vi "Execute.vi"(8 "error in (no error)":errorcluster, 10 "User Events in":refnum<class "User Events.lvclass">, 11 "Controller in":refnum<class "Controller.lvclass">) -> (0 "error out":errorcluster, 3 "Controller out":refnum<class "Controller.lvclass">)   [LabVIEW 2016, in "Controller.lvclass"]
uses:
  Controller.lvclass
  User Events/User Events.lvclass
  Typedefs/StateTypes.ctl
  User Events/User Events.lvclass/User Events.ctl
  Commands/Command/Command.lvclass
  Typedefs/HPMT_Typedefs.lvlib
  Model/Model/Model.lvclass
  Model/Boot Loader/Boot Loader.lvclass
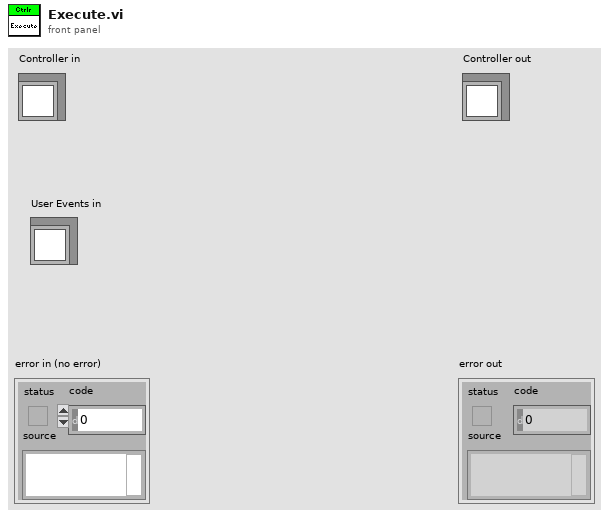
[diagram p1: front panel]
types:
  T1 = typedef "HPMT_Typedefs.lvlib/StateTypes.ctl" = enum16{"Offline State", "Fault State", "Standby State", "Disabled State", "Enabled State", "Wait For User Input State", "Test Actuator State", "Manual State"}
  T2 = typedef "HPMT_Typedefs.lvlib/Subscribe Data Events.ctl" = cluster{"Command":refnum<user-event>}
  T3 = typedef "HPMT_Typedefs.lvlib/Publish Data Events.ctl" = cluster{"State":refnum<user-event>, "ErrorCode":refnum<user-event>, "Scan Progress":refnum<user-event>, "All Test Status":refnum<user-event>, "ActuatorData":refnum<user-event>, "Test Settings":refnum<user-event>, "Stop Constant Query":refnum<user-event>}
  T4 = cluster{"Event Registration Refnum":refnum<event-registration>, "Event Registration Refnum":refnum<event-registration>}
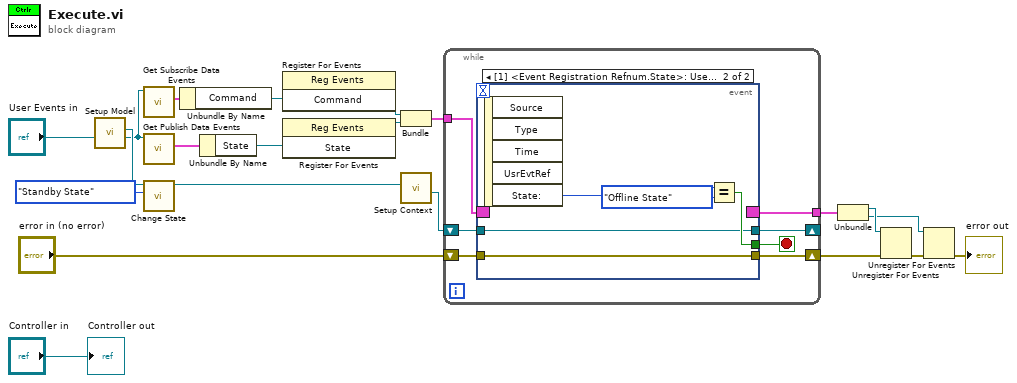
[diagram p0: block diagram]
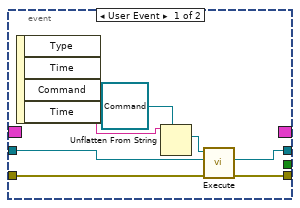
[diagram p2: hidden frame]
diagram:
  n1 = call "Setup Model.vi"("User Events in"="User Events in") -> ("User Events out"=w11:refnum<class "User Events.lvclass">, "Model out"=w16:refnum<class "Model.lvclass">)  [unwired: 7 in, 2 out]
  n2 = call "Get Subscribe Data Events.vi"("UserEvents in"=w11) -> ("Subscribe Data Events"=w20:T2)  [unwired: 9 in, 1 out]
  n3 = call "Get Publish Data Events.vi"("UserEvents in"=w11) -> ("Publish Data Events"=w10:T3)  [unwired: 9 in, 1 out]
  n4 = call "Change State.vi"("State Types"=StateTypes."Standby State" ("State:"), "Model in"=w16) -> ("Model out"=w15:refnum<class "Model.lvclass">)  [unwired: 8 in, 1 out]
  n5 = Unbundle By Name(w20) -> ("Command"=w18:refnum<user-event>)
  n6 = Unbundle By Name(w10) -> ("State"=w9:refnum<user-event>)
  n7 = register-events(w18) -> (reference out=w8:refnum<event-registration>)  [unwired: 2 in, 1 out]
  n8 = register-events(w9) -> (reference out=w7:refnum<event-registration>)  [unwired: 2 in, 1 out]
  n9 = Bundle("Event Registration Refnum"=w8, "Event Registration Refnum"=w7) -> (w6:T4)  [unwired: 1 in]
  n10 = call "Setup Context.vi"("Model in"=w15) -> ("Context out"=w14:refnum<class "Context.lvclass">)  [unwired: 8 in, 2 out]
  n11 = while {
    shift-right: [w27] -> w19
    shift-left: "error in (no error)" -> [w24]
    shift-right: [w26] -> _
    shift-left: w14 -> [w28]
    tunnel: w6 -> [w23]
    tunnel: [w22] -> w5
    stop <- w25 stop-if-true
    n12 = event shown="[1] <Event Registration Refnum.State>: User Event" {
      selector: w23 -> [_ _]
      dyn-events: [_ _] -> w22
      timeout: _ -> [_ _]
      tunnel: w28 -> [w33 w36]
      tunnel: [w32 w37] -> w27
      tunnel: [w31 w36] -> w26
      tunnel: [_ w38] -> w25
      tunnel: w24 -> [w30 w37]
      event User Event {
        n13 = event-data() -> ("Command"=w29:string)  [unwired: 1 in, 3 out]
        n14 = Unflatten From String(type=refnum<class "Command.lvclass"> refnum ("Command.lvclass"), binary string=w29) -> (value=w34:refnum<class "Command.lvclass">)  [unwired: 3 in, 2 out]
        n15 = call-dynamic "Execute.vi"("error in (no error)"=w30, "Context in"=w33, "Command in"=w34) -> ("error out"=w32:errorcluster, "Context out"=w31:refnum<class "Context.lvclass">)  [unwired: 6 in, 1 out]
      }
      event User Event {
        n16 = event-data() -> ("State:"=w40:T1)  [unwired: 1 in, 4 out]
        n17 = Equal?(x=w40, y=StateTypes."Offline State") -> (x = y?=w38:bool)
      }
    }
  }
  n18 = Unbundle(w5) -> ("Event Registration Refnum"=w4:refnum<event-registration>, "Event Registration Refnum"=w2:refnum<event-registration>)
  n19 = Unregister For Events(event registration refnum=w4, error in=w19) -> (error out=w3:errorcluster)
  n20 = Unregister For Events(event registration refnum=w2, error in=w3) -> (error out=→"error out":errorcluster)
  "Controller out" <- "Controller in"
